vi "修改类名.vi"() -> ()   [LabVIEW 2020]
panel:
  in  "VI路径":path
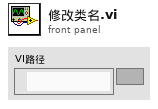
[diagram p1: front panel]
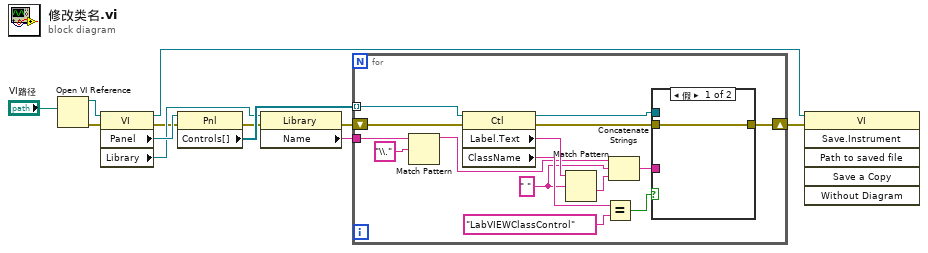
[diagram p0: block diagram]
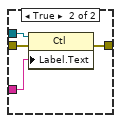
[diagram p2: hidden frame]
diagram:
  n1 = Open VI Reference(vi path="VI路径") -> (vi reference=w12:refnum<vi>, error out=w11:errorcluster)  [unwired: 5 in]
  n2 = property class="VI"(reference=w12, error in=w11) -> (reference out=w1:refnum<vi>, error out=w5:errorcluster, "Panel"=w10:refnum<vi>, "Library"=w8:refnum<vi>)
  n3 = property class="Pnl"(reference=w10, error in=w5) -> (error out=w4:errorcluster, "Controls[]"=w9:refnum<vi>[])  [unwired: 1 out]
  n4 = property class="Library"(reference=w8, error in=w4) -> (error out=w3:errorcluster, "Name"=w7:string)  [unwired: 1 out]
  n5 = for {
    tunnel: w9 -> [w27] mode=indexing
    tunnel: w7 -> [w20]
    shift-right: [w13] -> w2
    shift-left: w3 -> [w15]
    w18 = " " ("正则表达式")
    n6 = Match Pattern(string=w20, regular expression="\\." ("正则表达式")) -> (before substring=w19:string)  [unwired: 1 in, 3 out]
    n7 = property class="Ctl"(reference=w27, error in=w15) -> (reference out=w23:refnum<vi>, error out=w14:errorcluster, "Label.Text"=w22:string, "ClassName"=w26:string)
    n8 = Match Pattern(string=w22, regular expression=w18) -> (after substring=w17:string)  [unwired: 1 in, 3 out]
    n9 = Equal?(x=w26, y="LabVIEWClassControl") -> (x = y?=w24:bool)
    n10 = Concatenate Strings(w19, w18, w17) -> (w16:string)
    n11 = case shown="假" w24 {
      tunnel: w23 -> [_ w32]
      tunnel: w16 -> [_ w31]
      tunnel: w14 -> [w28 w30]
      tunnel: [w28 w29] -> w13
      frame False {
      }
      frame True {
        n12 = property class="Ctl"(reference=w32, error in=w30, "Label.Text"=w31) -> (error out=w29:errorcluster)  [unwired: 1 out]
      }
    }
  }
  n13 = invoke class="VI" method="Save.Instrument"(reference=w1, error in=w2) -> ()  [unwired: 4 in, 6 out]
